vi "Kinect - Hover (SubVI).vi"(8 "error in":errorcluster, 11 "Array of Joint Positions In":dbl[][](array[numeric])) -> (0 "error out":errorcluster, 2 "Boolean":bool, 3 "Array of Joint Positions Out":dbl[][](array[numeric]))   [LabVIEW 2014]
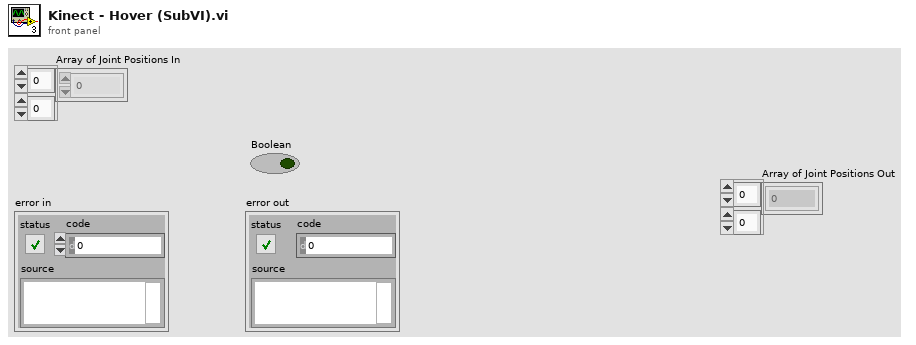
[diagram p1: front panel]
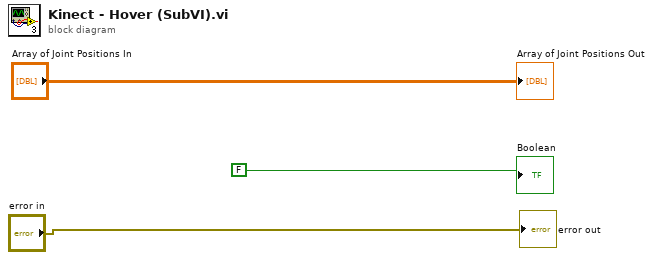
[diagram p0: block diagram]
diagram:
  "Boolean" <- FALSE
  "error out" <- "error in"
  "Array of Joint Positions Out" <- "Array of Joint Positions In"
